vi "mod_Find CPFSK Symbol Block Count.vi"() -> ()   [LabVIEW 2020, in "niDMT.lvlib"]
uses:
  <vilib>/addons/Modulation/niDMT.lvlib
  <vilib>/addons/Modulation/Digital/General/MT Generate FSK System Parameters(M).vi
panel:
  out "modulation index":dbl
  in  "frequency deviation":dbl
  in  "M-FSK (2)":i32=2
  in  "tolerance":dbl=1e-09
  out "Integer Multiple of 2*pi":dbl format="%.9g"
  out "Number of time (2^N-1) symbols to be repeated":i32
  in  "symbol rate":dbl
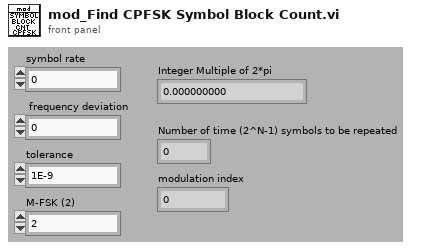
[diagram p1: front panel]
types:
  T1 = cluster{"samples per symbol (16)":i32, "symbol map":dbl[], "symbol phase continuity":enum16{"continuous", "discontinuous"}}
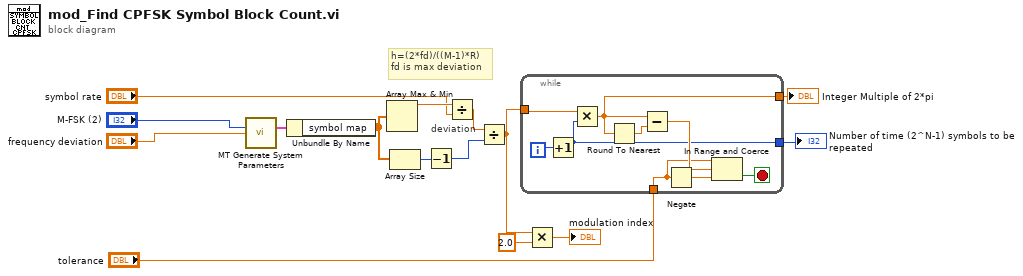
[diagram p0: block diagram]
diagram:
  # "h=(2*fd)/((M-1)*R)\nfd is max deviation"
  # "deviation"
  n1 = call-poly <vilib>:"MT Generate System Parameters.vi"("M-FSK (2)"="M-FSK (2)", "FSK deviation (Hz)"="frequency deviation") -> ("FSK system parameters"=w7:T1)  [unwired: 3 in, 10 out]
  n2 = Unbundle By Name(w7) -> ("symbol map"=w15:dbl[])
  n3 = Array Max & Min(array=w15) -> (max value=w11:dbl)  [unwired: 3 out]
  n4 = Array Size(array=w15) -> (size(s)=w14:i32)
  n5 = Decrement(x=w14) -> (x-1=w13:i32)
  n6 = Divide(x=w11, y="symbol rate") -> (x/y=w12:dbl)
  n7 = Divide(x=w12, y=w13) -> (x/y=w3:dbl)
  n8 = while {
    tunnel: w3 -> [w23]
    tunnel: [w18] -> w9
    tunnel: [w17] -> w10
    tunnel: "tolerance" -> [w16]
    i -> [w24]
    stop <- w19 stop-if-true
    n9 = Increment(x=w24) -> (x+1=w17:i32)
    n10 = Multiply(x=w23, y=w17) -> (x*y=w18:dbl)
    n11 = Round To Nearest(number=w18) -> (nearest integer value=w22:dbl)
    n12 = Subtract(x=w18, y=w22) -> (x-y=w21:dbl)
    n13 = Negate(x=w16) -> (-x=w20:dbl)
    n14 = In Range and Coerce(upper limit=w16, x=w21, lower limit=w20) -> (In Range?=w19:bool)  [unwired: 1 out]
  }
  "Number of time (2^N-1) symbols to be repeated" <- w10
  "Integer Multiple of 2*pi" <- w9
  n15 = Multiply(x=w3, y=2.0) -> (x*y=→"modulation index":dbl)
